vi "Time.vi"(1 "format":bool) -> (0 "Time":string)   [LabVIEW 2010]
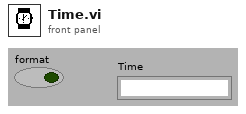
[diagram p1: front panel]
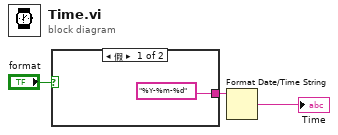
[diagram p0: block diagram]
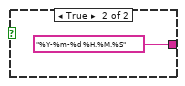
[diagram p2: hidden frame]
diagram:
  n1 = case shown="假" "format" {
    tunnel: ["%Y-%m-%d" ("time format string (%c)") "%Y-%m-%d %H.%M.%S" ("time format string (%c)")] -> w3
    frame False {
    }
    frame True {
    }
  }
  n2 = Format Date/Time String(time format string (%c)=w3) -> (date/time string=→"Time":string)  [unwired: 2 in]
